vi "Camera string test.vi"() -> ()   [LabVIEW 2018]
uses:
  <vilib>/myRIO/Instrument Drivers/Onboard IO/UART/typedef/VISA Configuration.ctl
  <vilib>/Instr/_visa.llb/VISA Configure Serial Port (Instr).vi
  <vilib>/myRIO/Express VI/Onboard IO/UART/UART Express VI.xnode
  <vilib>/vision/driver/NI_Vision_Acquisition_Software.lvlib
  <vilib>/myRIO/Instrument Drivers/Onboard IO/UART/UART.lvlib
panel:
  out "data string":string
  out "2D Picture":picture
  out "Pixels saved":i32
  out "Picture height":i32
  out "Picture width":i32
  out "Data String":string
  out "Image 5":T1(plugin-control)
  in  "Stop (F)":bool
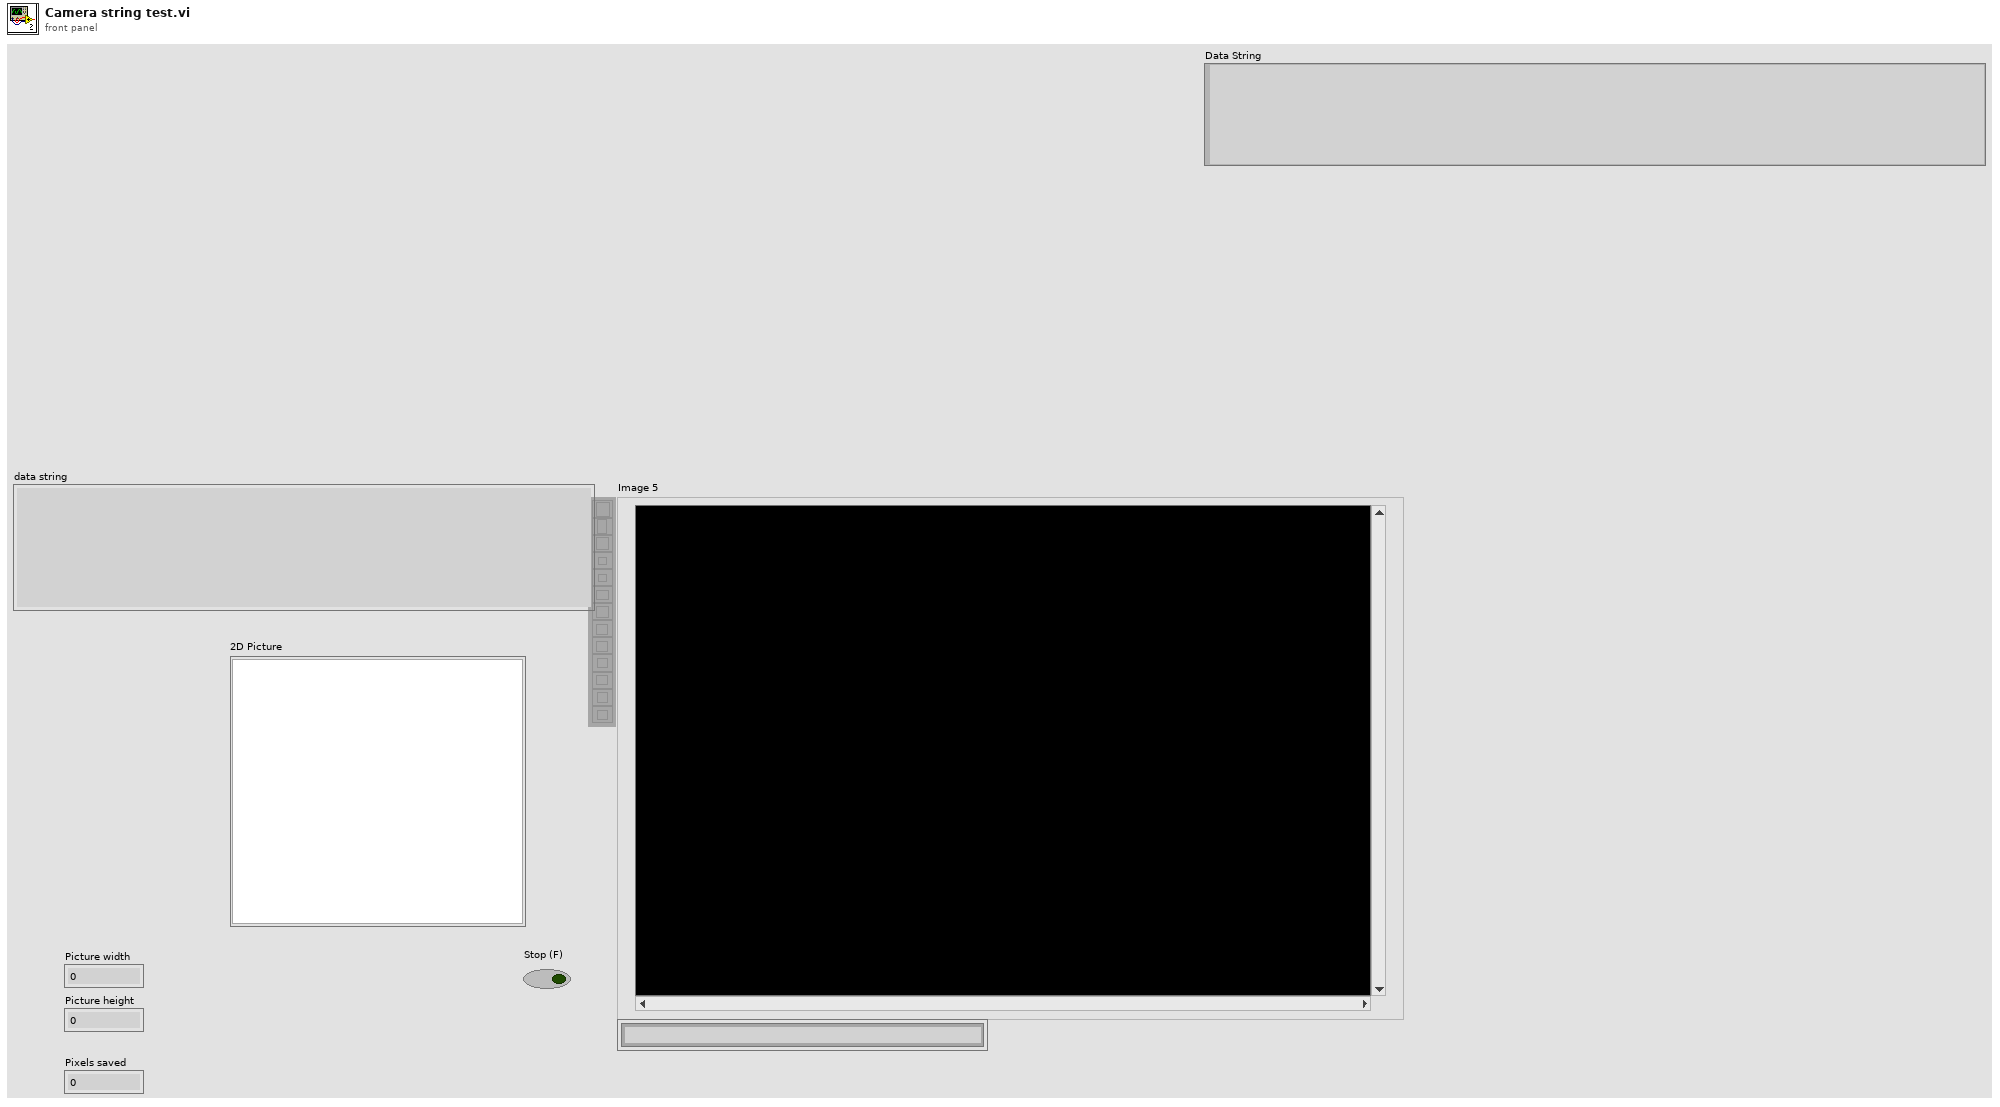
[diagram p1: front panel]
types:
  T1 = typedef "IMAQ Image.ctl" = refnum<image>
  T2 = typedef "UART.lvlib/VISA Configuration.ctl" = cluster{"baud rate (9600)":u32, "data bits (8)":u16, "parity (0:none)":enum16{"None", "Odd", "Even", "Mark", "Space"}, "stop bits (10: 1 bit)":u16, "flow control (0:none)":u16, "termination char\n(0xA = '\\n' = LF) ":u8, "Enable Termination\nChar (T)":bool, "timeout (10sec)":u32}
  T3 = typedef "IMAQdx.ctl" = refnum<k21>
  T4 = typedef "imagedata.ctl" = cluster{"image type":i32, "image depth":i32, "image":u8[], "mask":u8[], "colors":u32[], "Rectangle":cluster{"left":i16, "top":i16, "right":i16, "bottom":i16}}
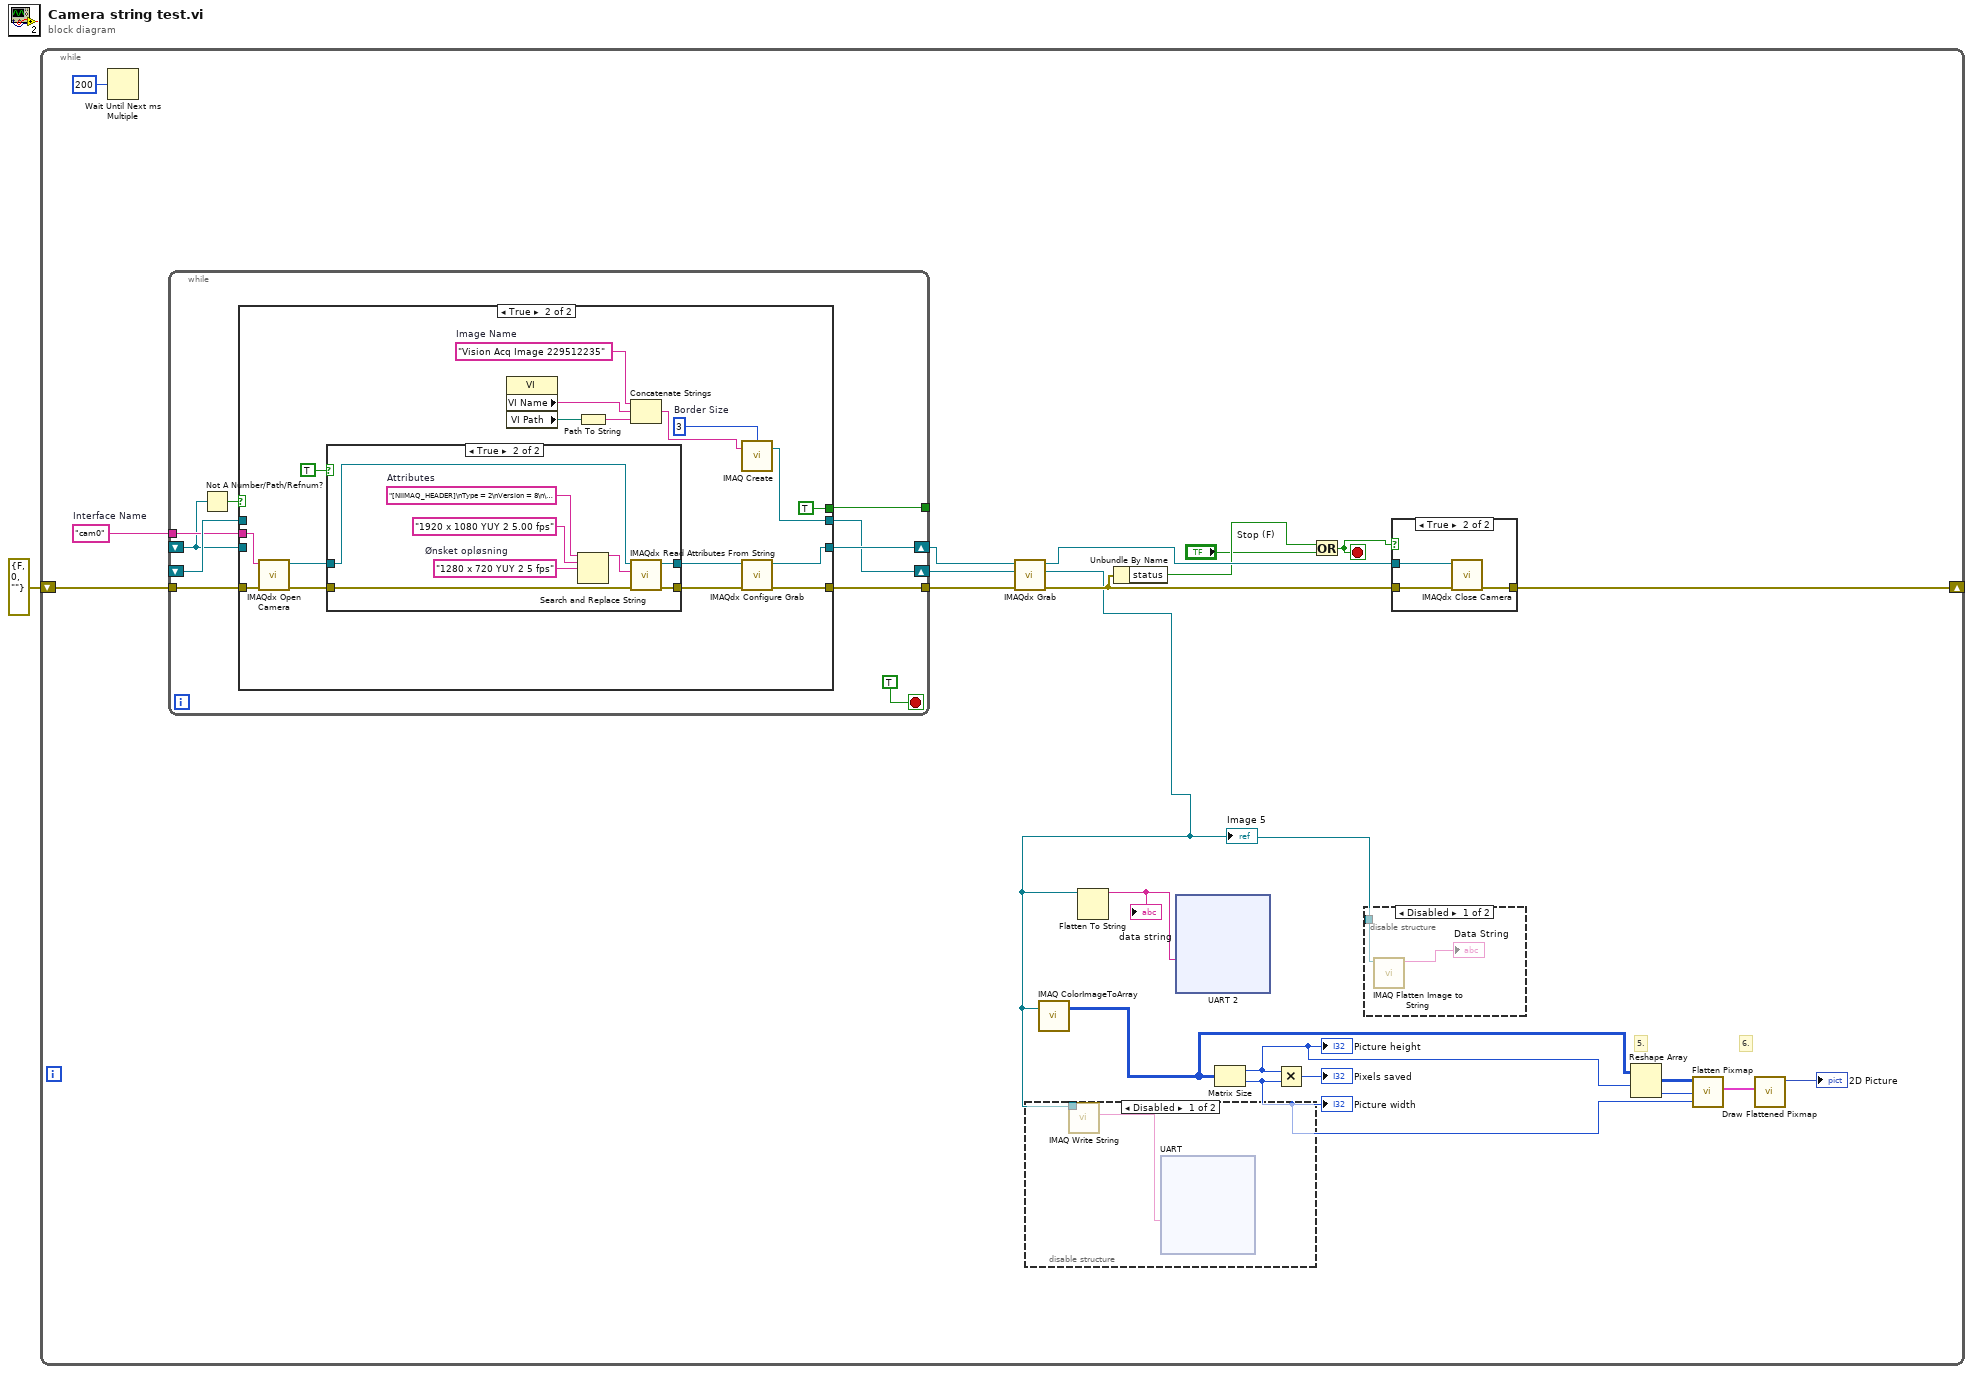
[diagram p0: block diagram]
diagram:
  n1 = while {
    shift-right: [w4] -> _
    shift-left: errorcluster {"status"=FALSE, "code"=0, "source"=""} ("error in") -> [w18]
    stop <- w20 stop-if-true
    w21 = "cam0"  # Interface Name
    # "6."
    # "5."
    n2 = Wait Until Next ms Multiple(millisecond multiple=u32 200) -> ()  [unwired: 1 out]
    n3 = while "While Loop_template0" {
      shift-right: [w72] -> w17
      shift-left: _ -> [w65]
      tunnel: [w71] -> w22
      tunnel: w18 -> [w70]
      shift-right: [w68] -> w16
      shift-left: _ -> [w67]
      tunnel: w21 -> [w66]
      tunnel: [w63] -> _
      stop <- TRUE ("_template0") stop-if-true
      n4 = Not A Number/Path/Refnum?(number/path/refnum=w65) -> (NaN/Path/Refnum?=w64:bool)
      n5 = case "Case Structure_template0" shown="True" w64 {
        tunnel: [w75 w91] -> w72
        tunnel: w65 -> [w75 _]
        tunnel: [w74 w90] -> w71
        tunnel: w70 -> [w74 w92]
        tunnel: [w73 w89] -> w68
        tunnel: w67 -> [w73 _]
        tunnel: w66 -> [_ w79]
        tunnel: [_ TRUE] -> w63
        frame False {
        }
        frame True {
          w76 = 3  # Border Size
          w84 = "Vision Acq Image 229512235"  # Image Name
          n6 = call <vilib>:"IMAQdx Open Camera.vi"("error in"=w92, "Session In"=w79) -> ("error out"=w82:errorcluster, "Session Out"=w83:T3)  [unwired: 1 in, 7 out]
          n7 = case shown="True" TRUE ("Init Attributes") {
            tunnel: w83 -> [w94 w102]
            tunnel: w82 -> [w93 w101]
            tunnel: [w94 w100] -> w81
            tunnel: [w93 w99] -> w80
            frame False {
            }
            frame True {
              w95 = "1280 x 720 YUY 2 5 fps"  # Ønsket opløsning
              w98 = "[NIIMAQ_HEADER]\nType = 2\nVersion = 8\n\n[CAMERA_DATA]\nAcquisitionAttributes::Bayer::Algorithm = \"Bilinear\"\nAcquisitionAttributes::Bayer::GainB = \"1\"\nAcquisitionAttributes::Bayer::GainG = \"1\"\nAcquisitionAttributes::Bayer::GainR = \"1\"\nAcquisitionAttributes::Bayer::Pattern = \"Use hardware value\"\nAcquisitionAttributes::BitsPerPixel = \"Use hardware value\"\nAcquisitionAttributes::HardwareMaximumQueuedBufferCount = \"1000\"\nAcquisitionAttributes::HardwareRequeueBufferListThreshold = \"50\"\nAcquisitionAttributes::IgnoreFirstFrame = \"false\"\nAcquisitionAttributes::ImageDecoderCopyMode = \"Auto\"\nAcquisitionAttributes::OutputImageType = \"Auto\"\nAcquisitionAttributes::OverwriteMode = \"Get Newest\"\nAcquisitionAttributes::PixelSignedness = \"Use hardware value\"\nAcquisitionAttributes::ReceiveTimestampMode = \"None\"\nAcquisitionAttributes::ShiftPixelBits = \"false\"\nAcquisitionAttributes::SwapPixelBytes = \"false\"\nAcquisitionAttributes::Timeout = \"5000\"\nAcquisitionAttributes::VideoMode = \"1920 x 1080 YUY 2 5.00 fps\"\nCameraAttributes::BacklightCompensation::Mode = \"Manual\"\nCameraAttributes::BacklightCompensation::Value = \"0\"\nCameraAttributes::Brightness::Mode = \"Manual\"\nCameraAttributes::Brightness::Value = \"168\"\nCameraAttributes::Contrast::Mode = \"Manual\"\nCameraAttributes::Contrast::Value = \"5\"\nCameraAttributes::Exposure::Mode = \"AutoAperaturePriority\"\nCameraAttributes::Focus::Mode = \"Auto\"\nCameraAttributes::Pan::Mode = \"Manual\"\nCameraAttributes::Pan::Value = \"0\"\nCameraAttributes::PowerLineFrequency::Mode = \"60Hz\"\nCameraAttributes::Saturation::Mode = \"Manual\"\nCameraAttributes::Saturation::Value = \"103\"\nCameraAttributes::Sharpness::Mode = \"Manual\"\nCameraAttributes::Sharpness::Value = \"25\"\nCameraAttributes::Tilt::Mode = \"Manual\"\nCameraAttributes::Tilt::Value = \"0\"\nCameraAttributes::WhiteBalance::Mode = \"Auto\"\nCameraAttributes::Zoom::Mode = \"Manual\"\nCameraAttributes::Zoom::Value = \"0\"\n"  # Attributes
              n8 = Search and Replace String(input string=w98, search string="1920 x 1080 YUY 2 5.00 fps", replace string=w95) -> (result string=w96:string)  [unwired: 5 in, 3 out]
              n9 = call <vilib>:"IMAQdx Read Attributes From String.vi"("error in"=w101, "Attributes String In"=w96, "Session In"=w102) -> ("error out"=w99:errorcluster, "Session Out"=w100:T3)  [unwired: 7 out]
            }
          }
          n10 = property class="VI"() -> ("VI Name"=w87:string, "VI Path"=w88:path)  [unwired: 2 in, 2 out]
          n11 = Path To String(path=w88) -> (string=w86:string)
          n12 = Concatenate Strings(w84, w87, w86) -> (w85:string)
          n13 = call "IMAQ Create"("Border Size"=w76, "Image Name"=w85) -> ("New Image"=w89:T1)  [unwired: 2 in, 2 out]
          n14 = call <vilib>:"IMAQdx Configure Grab.vi"("error in"=w80, "Session In"=w81) -> ("error out"=w90:errorcluster, "Session Out"=w91:T3)  [unwired: 8 out]
        }
      }
    }
    n15 = call <vilib>:"IMAQdx Grab.vi"("error in"=w22, "Image In"=w16, "Session In"=w17) -> ("error out"=w15:errorcluster, "Image Out"=w3:T1, "Session Out"=w14:T3)  [unwired: 1 in, 5 out]
    "Image 5" <- w3
    n16 = disable-structure shown="Disabled" {
      disable-tunnel: w3 -> [w40 _]
      frame Disabled {
        n17 = call-poly "IMAQ Write String"("Image"=w40) -> ("FileString"=w39:string)  [unwired: 8 in, 2 out]
        n18 = xnode "UART"("Characters to Write"=w39) -> ()  [unwired: 1 in, 2 out]
      }
      frame Enabled {
      }
    }
    n19 = call "IMAQ ColorImageToArray"("Image"=w3) -> ("Image Pixels (U32)"=w5:u32[][])  [unwired: 3 in, 2 out]
    n20 = Flatten To String(anything=w3) -> (data string=w2:string)  [unwired: 3 in, 2 out]
    "data string" <- w2
    n21 = Unbundle By Name(w15) -> ("status"=w13:bool)
    n22 = xnode "UART 2"("Characters to Write"=w2) -> ()  [unwired: 1 in, 2 out]
    n23 = Matrix Size(0:w5) -> (1:w6:i32, 2:w7:i32)
    "Picture width" <- w7
    "Picture height" <- w6
    n24 = Multiply(x=w6, y=w7) -> (x*y=→"Pixels saved":i32)
    n25 = Or(x=w13, y="Stop (F)") -> (x .or. y?=w20:bool)
    n26 = disable-structure shown="Disabled" {
      disable-tunnel: w3 -> [w58 _]
      frame Disabled {
        n27 = call "IMAQ Flatten Image to String"("Image"=w58) -> ("Data String"=→"Data String":string)  [unwired: 9 in, 1 out]
      }
      frame Enabled {
      }
    }
    n28 = case "Case Structure_template1" shown="True" w20 {
      tunnel: [w59 w61] -> w4
      tunnel: w15 -> [w59 w62]
      tunnel: w14 -> [_ w60]
      frame False {
      }
      frame True {
        n29 = call <vilib>:"IMAQdx Close Camera.vi"("error in"=w62, "Session In"=w60) -> ("error out"=w61:errorcluster)  [unwired: 9 out]
      }
    }
    n30 = Reshape Array(w5, w6, w7) -> (w8:u32[][])
    n31 = call <vilib>:"Flatten Pixmap.vi"("24-bit pixmap"=w8) -> ("image data"=w10:T4)  [unwired: 10 in]
    n32 = call <vilib>:"Draw Flattened Pixmap.vi"("image data"=w10) -> ("new picture"=→"2D Picture":picture)  [unwired: 8 in]
  }
